vi "Native Components.vi"(8 "error in (no error)":errorcluster) -> (0 "error out":errorcluster, 2 "native component names":string[](array[string]), 3 "native components":refnum<class>[](array[class]))   [LabVIEW 2017, in "DSF Core.lvlib"]
uses:
  DSF Core.lvlib
  Components/Buffer Converters/DSF Type Converter/DSF Type Converter.lvclass
  C:/Git/DSF/Core/Classes/Buffer Converter/Buffer Converter.lvclass
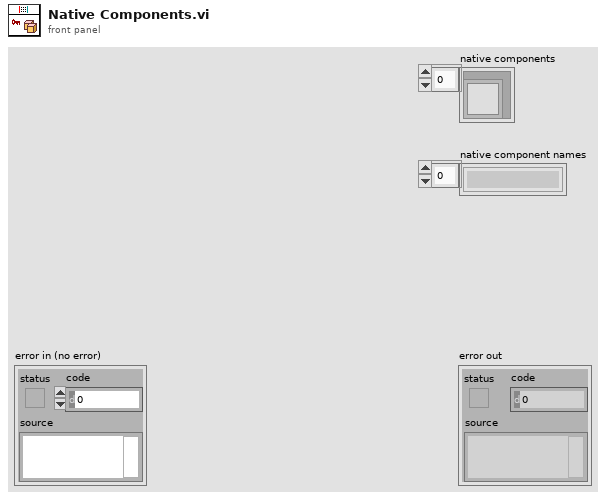
[diagram p1: front panel]
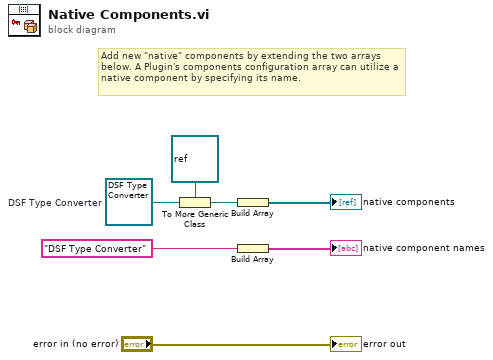
[diagram p0: block diagram]
diagram:
  w7 = refnum<class "DSF Type Converter.lvclass"> refnum  # DSF Type Converter
  # "Add new \"native\" components by extending the two arrays below. A Plugin's components configuration array can utilize a native component by specifying its name."
  n1 = To More Generic Class(target class=refnum<class> refnum ("LabVIEW Object"), reference=w7) -> (generic class reference=w6:refnum<class>)
  n2 = Build Array(w6) -> (→"native components":refnum<class>[])
  n3 = Build Array("DSF Type Converter") -> (→"native component names":string[])
  "error out" <- "error in (no error)"
